vi "Open System Definition.vi"(8 "error in (no error)":errorcluster, 11 "System Definition File":path) -> (0 "error out":errorcluster, 1 "Target Refnum":refnum<k24>, 2 "Root Refnum":refnum<k24>, 3 "System Definition Refnum":refnum<k24>)   [LabVIEW 2019]
uses:
  NationalInstruments.VeriStand.SystemDefinitionAPI
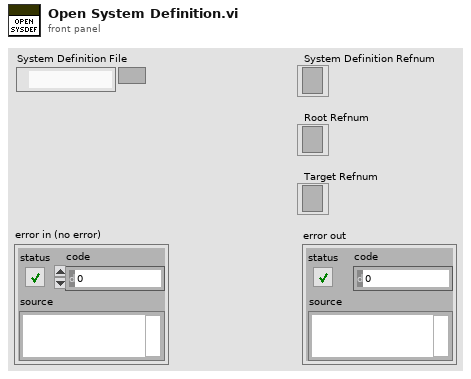
[diagram p1: front panel]
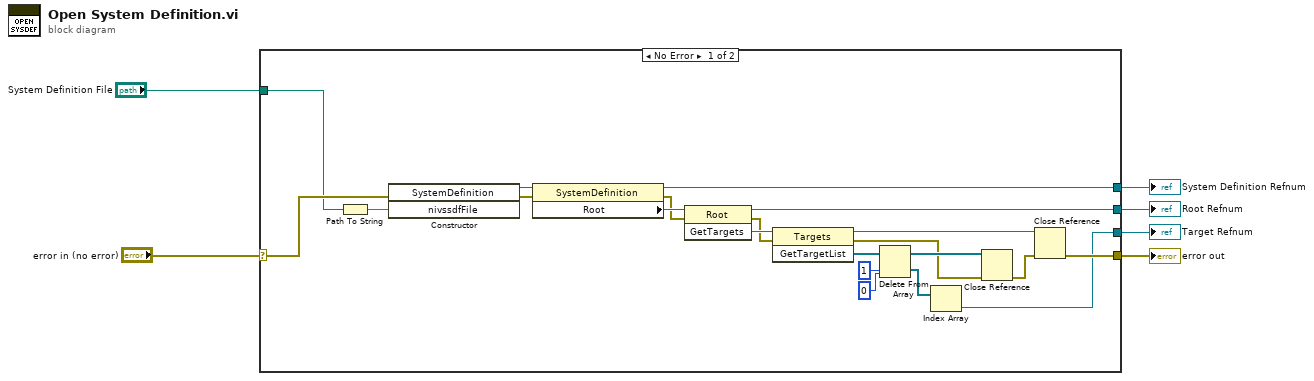
[diagram p0: block diagram]
diagram:
  n1 = case shown="No Error" "error in (no error)" {
    selector: "error in (no error)" -> [w12 w28]
    tunnel: [w11 w28] -> w5
    tunnel: "System Definition File" -> [w10 _]
    tunnel: [w9 _] -> w3
    tunnel: [w8 _] -> w2
    tunnel: [w7 _] -> w1
    frame No Error {
      n2 = Path To String(path=w10) -> (string=w13:string)
      n3 = constructor class="SystemDefinition"(error in=w12, "nivssdfFile"=w13) -> (reference out=w15:refnum<k24>, error out=w14:errorcluster)  [unwired: 2 in, 2 out]
      n4 = property class="SystemDefinition"(reference=w15, error in=w14) -> (reference out=w9:refnum<k24>, error out=w16:errorcluster, "Root"=w17:refnum<k24>)
      n5 = invoke class="Root" method="GetTargets"(reference=w17, error in=w16) -> (reference out=w8:refnum<k24>, error out=w18:errorcluster, "GetTargets"=w19:refnum<k24>)  [unwired: 1 in]
      n6 = invoke class="Targets" method="GetTargetList"(reference=w19, error in=w18) -> (reference out=w26:refnum<k24>, error out=w23:errorcluster, "GetTargetList"=w20:refnum<k24>[])  [unwired: 1 in]
      n7 = Delete From Array(array=w20, length=1, index=0) -> (deleted portion=w27:refnum<k24>[], array with subset deleted=w24:refnum<k24>[])
      n8 = Index Array(array=w27) -> (element=w7:refnum<k24>)  [unwired: 1 in]
      n9 = Close Reference(reference=w24, error in (no error)=w23) -> (error out=w25:errorcluster)
      n10 = Close Reference(reference=w26, error in (no error)=w25) -> (error out=w11:errorcluster)
    }
    frame Error {
    }
  }
  "error out" <- w5
  "Root Refnum" <- w2
  "System Definition Refnum" <- w3
  "Target Refnum" <- w1
